vi "VisionAlign.vi"() -> (0 "Z":dbl, 2 "Y":dbl, 3 "X":dbl)   [LabVIEW 2018]
uses:
  <vilib>/Rock Robotics/Network Tables/NT Read Numeric Array.vi
  Globals.vi
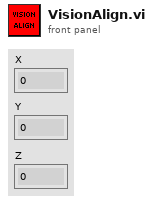
[diagram p1: front panel]
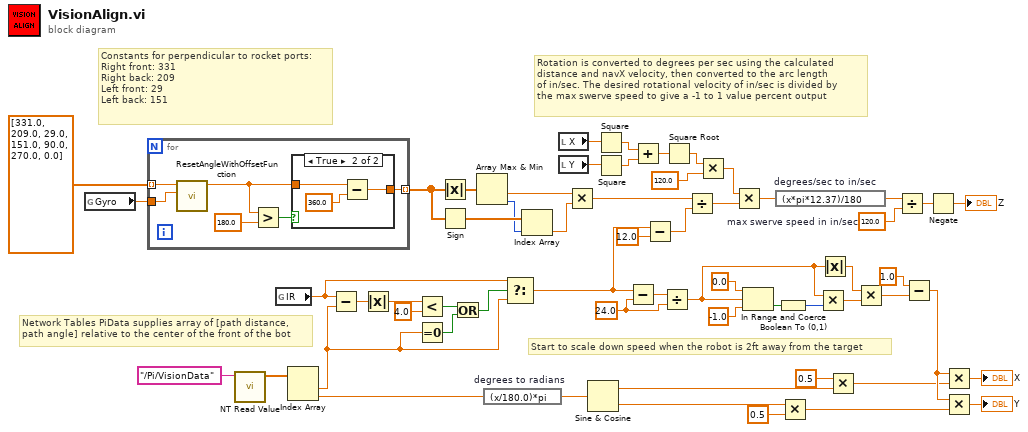
[diagram p0: block diagram]
diagram:
  w11 = 120.0  # max swerve speed in in/sec
  w29 = 24.0 ("y")
  # "Start to scale down speed when the robot is 2ft away from the target"
  # "Rotation is converted to degrees per sec using the calculated\ndistance and navX velocity, then converted to the arc length\nof in/sec. The desired rotational velocity of in/sec is divided by\nthe max swerve speed to give a -1 to 1 value percent output"
  # "Network Tables PiData supplies array of [path distance,\npath angle] relative to the center of the front of the bot"
  # "Constants for perpendicular to rocket ports:\nRight front: 331\nRight back: 209\nLeft front: 29\nLeft back: 151"
  n1 = global read "Globals.vi" "Gyro"() -> (w56:dbl)
  n2 = for {
    tunnel: dbl[] [331.0, 209.0, 29.0, 151.0, 90.0, 270.0, 0.0] -> [w64] mode=indexing
    tunnel: w56 -> [w63]
    tunnel: [w62] -> w50 mode=indexing
    n3 = call "ResetAngleWithOffsetFunction.vi"("Offset"=w63, "AngleInput"=w64) -> ("AngleOutput"=w61:dbl)  [unwired: 9 in]
    n4 = Greater?(x=w61, y=180.0) -> (0:w59:bool)
    n5 = case shown="True" w59 {
      tunnel: w61 -> [w65 w67]
      tunnel: [w65 w66] -> w62
      frame False {
      }
      frame True {
        n6 = Subtract(x=w67, y=360.0) -> (x-y=w66:dbl)
      }
    }
  }
  n7 = call-poly <vilib>:"NT Read Value.vi"("Name"="/Pi/VisionData" ("Client Name")) -> ("Numeric Array"=w57:dbl[])  [unwired: 9 in, 1 out]
  n8 = global read "Globals.vi" "IR"() -> (w42:dbl)
  n9 = Index Array(array=w57) -> (element #1=w39:dbl, element #2=w26:dbl)  [unwired: 2 in]
  n10 = Subtract(x=w42, y=w39) -> (x-y=w44:dbl)
  n11 = Absolute Value(x=w44) -> (abs(x)=w24:dbl)
  n12 = Less?(x=w24, y=4.0) -> (x < y?=w43:bool)
  n13 = Equal To 0?(x=w39) -> (x = 0?=w40:bool)
  n14 = Absolute Value(x=w50) -> (abs(x)=w53:dbl[])
  n15 = Sign(1:w50) -> (0:w49:dbl[])
  n16 = Or(x=w43, y=w40) -> (x .or. y?=w41:bool)
  n17 = Array Max & Min(array=w53) -> (min value=w52:dbl, min index (indices)=w45:i32)  [unwired: 2 out]
  n18 = expression code="(x/180.0)*pi" "degrees to radians"(w26) -> (w55:dbl)
  n19 = Select(t=w42, s=w41, f=w39) -> (s? t:f=w38:dbl)
  n20 = Index Array(array=w49, index=w45) -> (element=w48:dbl)
  n21 = local read "X"() -> (w8:dbl)
  n22 = local read "Y"() -> (w7:dbl)
  n23 = Multiply(x=w52, y=w48) -> (x*y=w51:dbl)
  n24 = Sine & Cosine(0:w55) -> (1:w25:dbl, 2:w16:dbl)
  n25 = Square(x=w8) -> (x^2=w6:dbl)
  n26 = Square(x=w7) -> (x^2=w5:dbl)
  n27 = Subtract(x=w38, y=w29) -> (x-y=w37:dbl)
  n28 = Add(x=w6, y=w5) -> (x+y=w4:dbl)
  n29 = Subtract(x=w38, y=12.0) -> (x-y=w46:dbl)
  n30 = Divide(x=w37, y=w29) -> (x/y=w31:dbl)
  n31 = Square Root(x=w4) -> (sqrt(x)=w3:dbl)
  n32 = Divide(x=w51, y=w46) -> (x/y=w14:dbl)
  n33 = Multiply(x=w3, y=120.0) -> (x*y=w1:dbl)
  n34 = Multiply(x=w1, y=w14) -> (x*y=w13:dbl)
  n35 = In Range and Coerce(upper limit=0.0, x=w31, lower limit=-1.0) -> (In Range?=w34:bool)  [unwired: 1 out]
  n36 = expression code="(x*pi*12.37)/180" "degrees/sec to in/sec"(w13) -> (w12:dbl)
  n37 = Boolean To (0,1)(Boolean=w34) -> (0, 1=w33:i16)
  n38 = Multiply(x=w16, y=0.5) -> (x*y=w17:dbl)
  n39 = Multiply(x=w31, y=w33) -> (x*y=w32:dbl)
  n40 = Absolute Value(x=w31) -> (abs(x)=w30:dbl)
  n41 = Multiply(x=0.5, y=w25) -> (x*y=w19:dbl)
  n42 = Multiply(x=w30, y=w32) -> (x*y=w22:dbl)
  n43 = Divide(x=w12, y=w11) -> (x/y=w10:dbl)
  n44 = Subtract(x=1.0, y=w22) -> (x-y=w21:dbl)
  n45 = Negate(x=w10) -> (-x=→"Z":dbl)
  n46 = Multiply(x=w21, y=w19) -> (x*y=→"X":dbl)
  n47 = Multiply(x=w21, y=w17) -> (x*y=→"Y":dbl)
